vi "timertest.vi"() -> ()   [LabVIEW 2017]
panel:
  in  "stop":bool
  in  "OK Button":bool
  out "Numeric":dbl
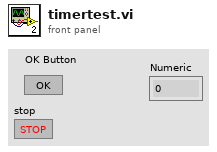
[diagram p1: front panel]
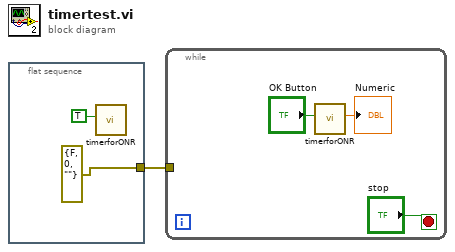
[diagram p0: block diagram]
diagram:
  n1 = flat-sequence {
    tunnel: [errorcluster {"status"=FALSE, "code"=0, "source"=""} ("error constant")] -> w1
    frame #0 {
      n2 = call "timerforONR.vi"("Boolean"=TRUE) -> ()  [unwired: 10 in, 1 out]
    }
  }
  n3 = while {
    tunnel: w1 -> [_]
    stop <- "stop" stop-if-true
    n4 = call "timerforONR.vi"("Boolean"="OK Button") -> ("Numeric"=→"Numeric":dbl)  [unwired: 10 in]
  }
